vi "save operation binary.vi"(8 "error in":errorcluster, 11 "state cluster":T1) -> (0 "error out":errorcluster, 3 "state out":T1)   [LabVIEW 2013, in "Standard Editor.lvlib"]
uses:
  Standard Editor.lvlib
  Controls/StateCluster.ctl
  Configuration Editor/Classes/SystemConfigRepo/SystemConfigRepo.lvclass
  Configuration Editor/Classes/Systems/Systems.lvclass
  <vilib>/NI/Configuration Framework/Node/StandardEvents.ctl
  <vilib>/NI/Configuration Framework/Node/UserEventRef.ctl
  <vilib>/NI/Configuration Framework/Controls/EventCluster.ctl
  <vilib>/NI/Configuration Framework/Node/NodeChangeEvent.ctl
  <vilib>/NI/Configuration Framework/Node/NodeRef.ctl
  <vilib>/NI/Configuration Framework/Node/NISE_CEF_Node.lvclass
  <vilib>/NI/Configuration Framework/Node/CacheState.ctl
  <vilib>/NI/Configuration Framework/Node/RefreshUIEvent.ctl
  <vilib>/NI/Configuration Framework/Node/StopEvent.ctl
  <vilib>/NI/Configuration Framework/glyph manager/glyph manager.ctl
  <vilib>/picture/picture.llb/imagedata.ctl
  <vilib>/NI/AMC/Message Queue.ctl
  <vilib>/NI/AMC/Message.ctl
  <vilib>/NI/Tools/Keyed Array/KeyedArray.ctl
  <vilib>/NI/Configuration Framework/hierarchy repo/NISE_CEF_HierarchyRepo.lvclass
  <vilib>/NI/Configuration Framework/tree serializer/NISE_CEF_TreeSerializer.lvlib
  <vilib>/NI/Configuration Framework/NISE_CEF_TreeControl.lvlib
  <vilib>/NI/Configuration Framework/glyph manager/glyph manager.lvlib
  <vilib>/NI/Tools/Keyed Array/Tools_KeyedArray.lvlib
  <vilib>/NI/AMC/AMC.lvlib
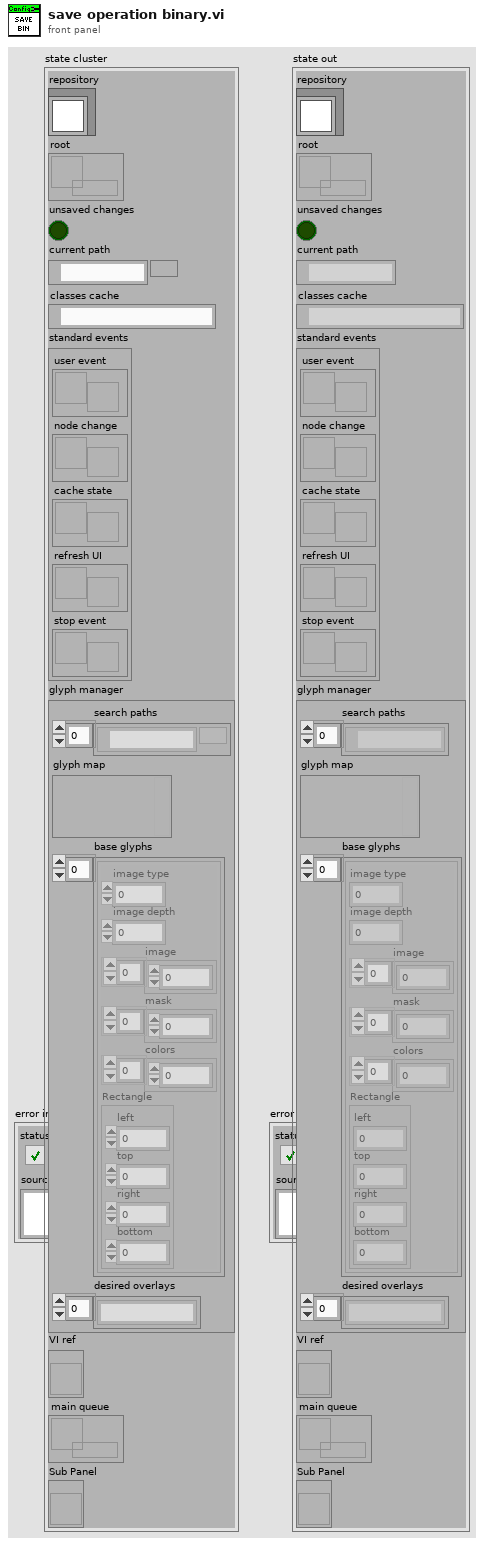
[diagram p1: front panel]
types:
  T1 = typedef "Standard Editor.lvlib/StateCluster.ctl" = cluster{"repository":refnum<class "SystemConfigRepo.lvclass">, "root":refnum<data-value>, "unsaved changes":bool, "current path":path, "classes cache":path, "standard events":T2, "glyph manager":T8, "VI ref":refnum<vi>, "main queue":T10, "Sub Panel":refnum<vi>}
  T2 = typedef "NISE_CEF_Node.lvclass/StandardEvents.ctl" = cluster{"user event":T3, "node change":T4, "cache state":T5, "refresh UI":T6, "stop event":T7}
  T3 = typedef "NISE_CEF_Node.lvclass/UserEventRef.ctl" = refnum<user-event>
  T4 = typedef "NISE_CEF_Node.lvclass/NodeChangeEvent.ctl" = refnum<user-event>
  T5 = typedef "NISE_CEF_Node.lvclass/CacheState.ctl" = refnum<user-event>
  T6 = typedef "NISE_CEF_Node.lvclass/RefreshUIEvent.ctl" = refnum<user-event>
  T7 = typedef "NISE_CEF_Node.lvclass/StopEvent.ctl" = refnum<user-event>
  T8 = typedef "glyph manager.lvlib/glyph manager.ctl" = cluster{"search paths":path[], "glyph map":variant, "base glyphs":T9[], "desired overlays":string[]}
  T9 = typedef "imagedata.ctl" = cluster{"image type":i32, "image depth":i32, "image":u8[], "mask":u8[], "colors":u32[], "Rectangle":cluster{"left":i16, "top":i16, "right":i16, "bottom":i16}}
  T10 = typedef "AMC.lvlib/Message Queue.ctl" = refnum<queue>
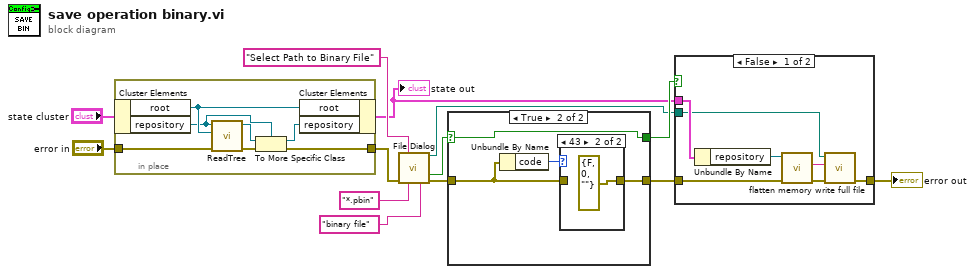
[diagram p0: block diagram]
diagram:
  n1 = in-place {
    in-place-border: "error in" -> [w20]
    in-place-border: [w17] -> w13
    n2 = in-place-cluster #1("state cluster") -> ("root"=w19:refnum<data-value>, "repository"=w15:refnum<class "SystemConfigRepo.lvclass">)
    n3 = call-dynamic "ReadTree.vi"("error in"=w20, "root"=w19, "repository in"=w15) -> ("error out"=w18:errorcluster, "repository out"=w16:refnum<class "NISE_CEF_Repository.lvclass">)  [unwired: 7 in]
    n4 = To More Specific Class(target class=w15, reference=w16, error in=w18) -> (specific class reference=w14:refnum<class "SystemConfigRepo.lvclass">, error out=w17:errorcluster)
    n5 = in-place-cluster #1("root"=w19, "repository"=w14) -> (w1:T1)
  }
  "state out" <- w1
  n6 = call "File Dialog"("prompt"="Select Path to Binary File" ("Prompt"), "error in"=w13, "pattern (all files)"="*.pbin" ("pattern"), "pattern label"="binary file") -> ("selected path"=w8:path, "cancelled"=w3:bool, "error out"=w2:errorcluster)  [unwired: 8 in, 1 out]
  n7 = case shown="True" w3 {
    selector: w3 -> [w21 w23]
    tunnel: w2 -> [w22 w25]
    tunnel: [w22 w24] -> w7
    tunnel: [w21 w23] -> w9
    frame False {
    }
    frame True {
      n8 = Unbundle By Name(w25) -> ("code"=w26:i32)
      n9 = case shown="43" w26 {
        tunnel: w25 -> [w27 _]
        tunnel: [w27 errorcluster {"status"=FALSE, "code"=0, "source"=""} ("error out")] -> w24
        frame Default {
        }
        frame 43 {
        }
      }
    }
  }
  n10 = case shown="False" w9 {
    tunnel: w1 -> [w35 _]
    tunnel: w7 -> [w32 w36]
    tunnel: [w29 w36] -> w12
    tunnel: w8 -> [w31 _]
    frame False {
      n11 = Unbundle By Name(w35) -> ("repository"=w33:refnum<class "SystemConfigRepo.lvclass">)
      n12 = call <vilib>:"flatten memory.vi"("error in"=w32, "NISE_CEF_HierarchyRepo in"=w33) -> ("error out"=w30:errorcluster, "binary repo"=w34:string)  [unwired: 7 in, 1 out]
      n13 = call <vilib>:"write full file.vi"("error in"=w30, "strings"=w34, "file path"=w31) -> ("error out"=w29:errorcluster)  [unwired: 8 in]
    }
    frame True {
    }
  }
  "error out" <- w12
